vi "Filter value to string.vi"(9 "filter set":T1) -> (10 "filter string":string)   [LabVIEW 2011]
uses:
  filter.ctl
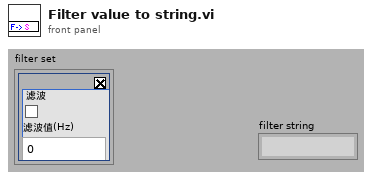
[diagram p1: front panel]
types:
  T1 = typedef "filter.ctl" = cluster{"en":bool, "value":i32, "Boolean":bool}
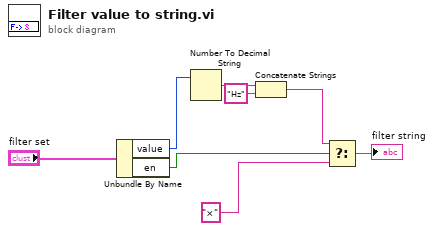
[diagram p0: block diagram]
diagram:
  n1 = Unbundle By Name("filter set") -> ("value"=w5:i32, "en"=w7:bool)
  n2 = Number To Decimal String(number=w5) -> (decimal integer string=w4:string)  [unwired: 1 out]
  n3 = Concatenate Strings(w4, "Hz" ("string")) -> (w2:string)
  n4 = Select(t=w2, s=w7, f="×") -> (s? t:f=→"filter string":string)
